vi "LV_to_int_time.vi"(7 "error in (no error)":errorcluster, 10 "Time Stamp":timestamp) -> (0 "error out":errorcluster, 3 "Integer Time":i64)   [LabVIEW 2013]
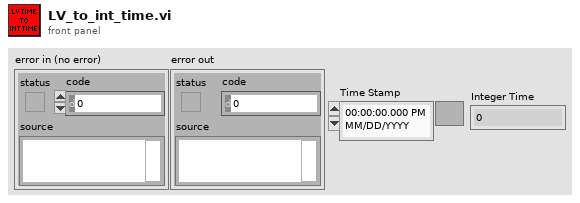
[diagram p1: front panel]
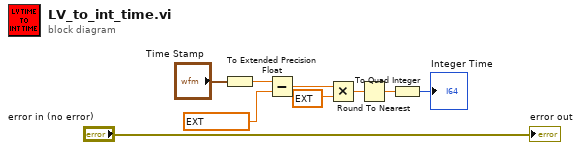
[diagram p0: block diagram]
diagram:
  n1 = To Extended Precision Float(1:"Time Stamp") -> (0:w1:ext)
  n2 = Subtract(x=w1, y=ext 2082844800.0) -> (x-y=w7:ext)
  n3 = Multiply(x=w7, y=ext 1000.0) -> (x*y=w4:ext)
  n4 = Round To Nearest(number=w4) -> (nearest integer value=w3:ext)
  n5 = To Quad Integer(1:w3) -> (0:→"Integer Time":i64)
  "error out" <- "error in (no error)"
